vi "lab7.vi"() -> ()   [LabVIEW 2020]
uses:
  <vilib>/measure/NI_MABase.lvlib
  <vilib>/measure/NI_MAPro.lvlib
  <vilib>/gmath/NI_Gmath.lvlib
  <vilib>/Analysis/NI_AALPro.lvlib
  <vilib>/Analysis/2dsp.llb/Power Spectrum (DBL).vi
  <vilib>/Analysis/4window.llb/Blackman Window (DBL).vi
  <vilib>/measure/macond.llb/IIR Filter for 1 Chan.vi
  <vilib>/Analysis/4window.llb/Cosine Tapered Window (DBL).vi
  <vilib>/Analysis/4window.llb/Hamming Window (DBL).vi
  <vilib>/Analysis/4window.llb/Blackman-Harris Window (DBL).vi
  <vilib>/Analysis/3filter.llb/Filter Structure Type.ctl
  <vilib>/Analysis/NI_AALBase.lvlib
panel:
  in  "OK Button":bool
  in  "signal type 2":T1(ring)
  out "Intensity Chart":sgl[][](graph)
  out "Waveform Chart 2":dbl[](graph)
  out "Waveform Chart":dbl[](graph)
  in  "?":bool
  in  "Amplitude 4":dbl=1.0 format="%.2p"
  in  "Window type 2":T2(ring)
  in  "filter structure option 2":T3=10 items=["IIR 2nd Order"=0, "IIR 4th Order"=1, "Auto Select"=10]
  in  "Filter specifications 2":T4={"Topology"=enum."Butterworth", "Type"=enum."Lowpass", "Order"=1, "Lower Fc"=100.0, "Upper Fc"=200.0, "PB Ripple"=1.0, "SB Attenuation"=60.0} {"PB Ripple" format="%0.2f"; "SB Attenuation" format="%0.2f"; "Lower Fc" format="%0.2p"; "Upper Fc" format="%0.2p"}
  out "Filtered 2":waveform(dbl)(graph)
  out "Sig + noise 2":waveform(dbl)(graph)
  in  "Reset Noise 2":bool
  out "Noise 2":waveform(dbl)(graph)
  in  "noise type 2":T5(ring)
  in  "Mean 2":dbl
  in  "Order 2":dbl
  in  "Start freq 2":dbl
  in  "Delta freq 2":dbl
  in  "Amplitude 2":dbl
  out "Signal 2":waveform(dbl)(graph)
  in  "Reset 2":bool
  in  "Offset 2":dbl
  in  "Square duty cycle, %  2":dbl
  in  "Amplitude 3":dbl
  in  "Phase 2":dbl
  in  "Frequncy 2":dbl
  in  "?":T6(tab)
  # "Sine Wave parameters"
  # "Gamma noise parameters"
  # "Poisson noise parameters"
  # "Other Wave-types parameters"
  # "Multitone noise parameters"
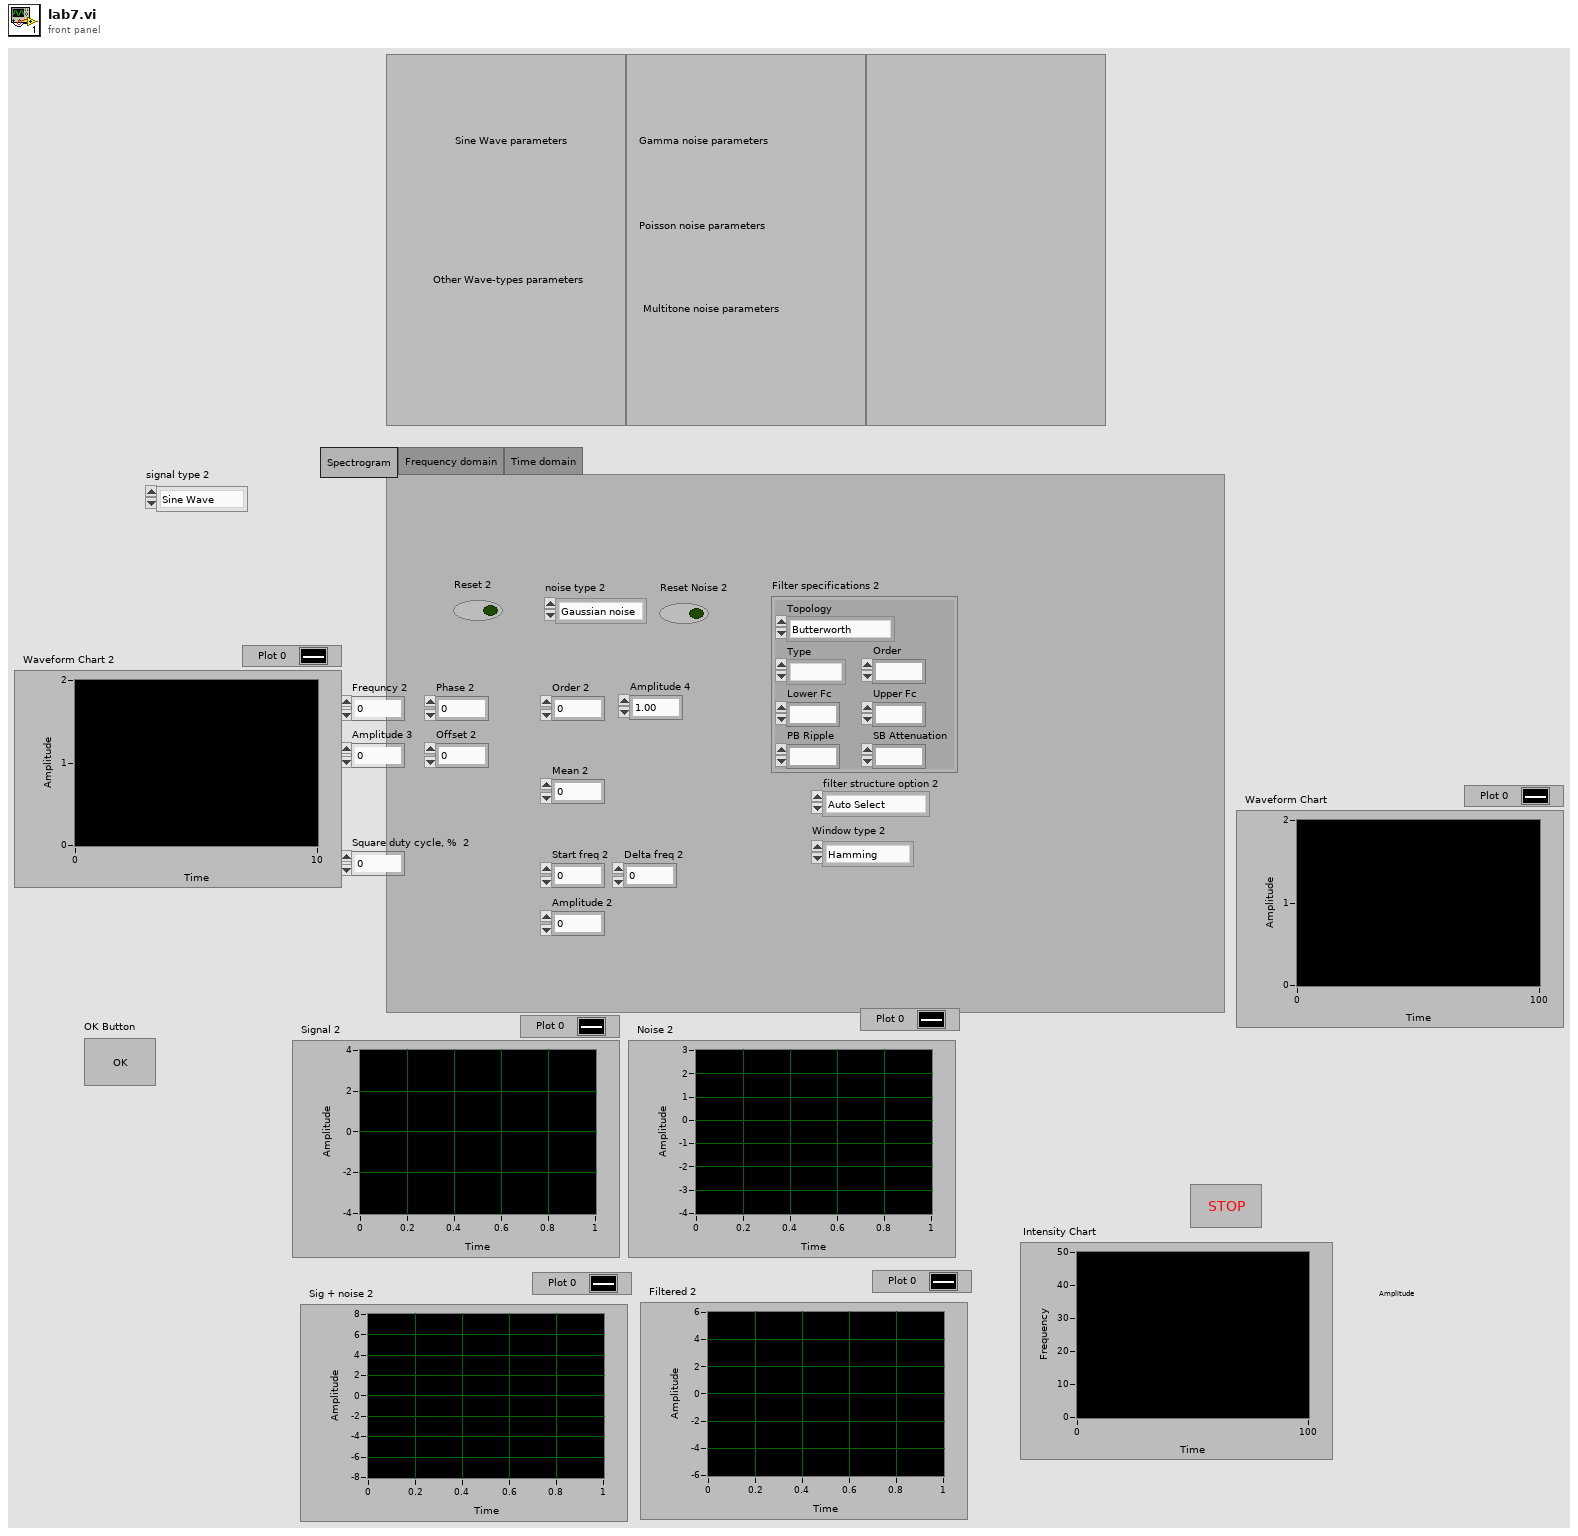
[diagram p1: front panel]
types:
  T1 = enum16{"Sine Wave", "Triangle Wave", "Square Wave", "Sawtooth Wave"}
  T2 = enum16{"Hamming", "Blackman", "Blackman-Harris", "Tapered cos"}
  T3 = typedef "NI_AALBase.lvlib/Filter Structure Type.ctl" = u16
  T4 = cluster{"Topology":enum16{"Off", "Butterworth", "Chebyshev", "Inverse Chebyshev", "Elliptic", "Bessel"}, "Type":enum16{"Lowpass", "Highpass", "Bandpass", "Bandstop"}, "Order":i32, "Lower Fc":dbl, "Upper Fc":dbl, "PB Ripple":dbl, "SB Attenuation":dbl}
  T5 = enum16{"Gaussian noise", "Multitone Noise", "Gamma Noise", "Poisson Noise"}
  T6 = enum32{"Spectrogram", "Frequency domain", "Time domain"}
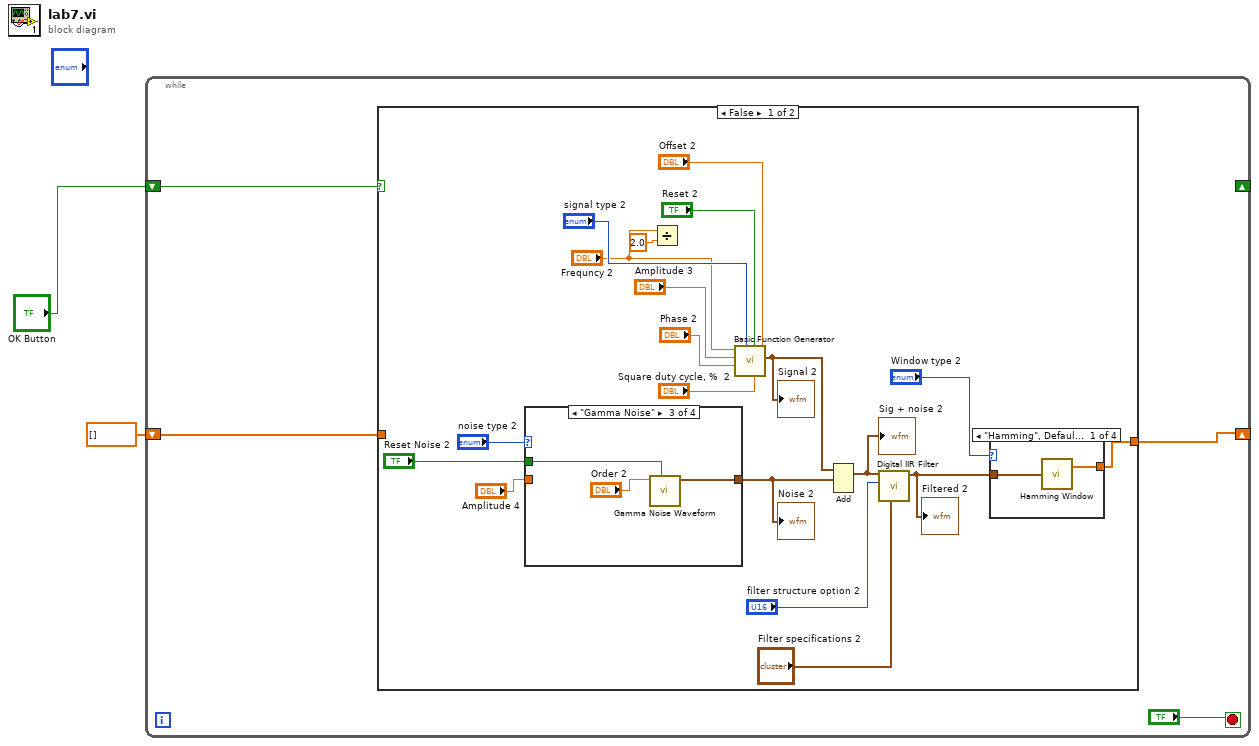
[diagram p0: block diagram]
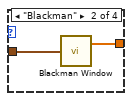
[diagram p2: hidden frame]
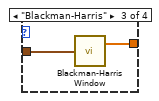
[diagram p3: hidden frame]
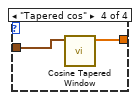
[diagram p4: hidden frame]
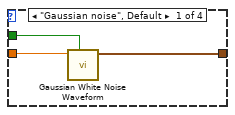
[diagram p5: hidden frame]
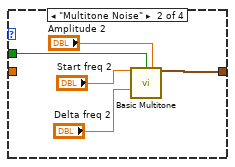
[diagram p6: hidden frame]
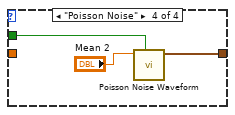
[diagram p7: hidden frame]
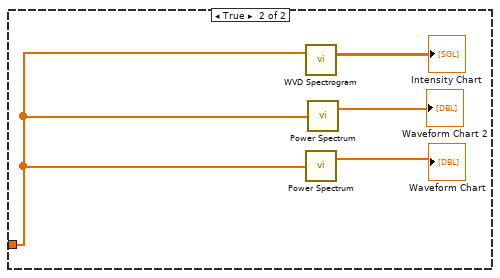
[diagram p8: hidden frame]
diagram:
  n1 = while {
    shift-right: [w4] -> _
    shift-left: dbl[] [] ("Windowed X") -> [w5]
    shift-right: _ -> [_]
    shift-left: "OK Button" -> [w3]
    stop <- "?" stop-if-true
    n2 = case shown="False" w3 {
      tunnel: [w7 _] -> w4
      tunnel: w5 -> [_ w49]
      frame False {
        n3 = case shown="\"Gamma Noise\"" "noise type 2" {
          tunnel: [w36 w40 w43 w45] -> w15
          tunnel: "Reset Noise 2" -> [w35 w41 w42 w47]
          tunnel: "Amplitude 4" -> [w34 _ _ _]
          frame "Gaussian noise", Default {
            n4 = call <vilib>:"Gaussian White Noise Waveform.vi"("reset signal"=w35, "standard deviation"=w34) -> ("signal out"=w36:waveform(dbl))  [unwired: 8 in, 1 out]
          }
          frame "Multitone Noise" {
            n5 = call <vilib>:"Basic Multitone.vi"("start frequency"="Start freq 2", "reset signal"=w41, "amplitude"="Amplitude 2", "delta frequency"="Delta freq 2") -> ("signal out"=w40:waveform(dbl))  [unwired: 8 in, 3 out]
          }
          frame "Gamma Noise" {
            n6 = call <vilib>:"Gamma Noise Waveform.vi"("reset signal"=w42, "order"="Order 2") -> ("signal out"=w43:waveform(dbl))  [unwired: 8 in, 1 out]
          }
          frame "Poisson Noise" {
            n7 = call <vilib>:"Poisson Noise Waveform.vi"("reset signal"=w47, "mean"="Mean 2") -> ("signal out"=w45:waveform(dbl))  [unwired: 8 in, 1 out]
          }
        }
        "Noise 2" <- w15
        n8 = Divide(x="Frequncy 2", y=2.0) -> ()  [unwired: 1 out]
        n9 = call <vilib>:"Basic Function Generator.vi"("offset"="Offset 2", "square wave duty cycle (%)"="Square duty cycle, %  2", "reset signal"="Reset 2", "signal type"="signal type 2", "phase"="Phase 2", "amplitude"="Amplitude 3", "frequency"="Frequncy 2") -> ("signal out"=w12:waveform(dbl))  [unwired: 2 in, 2 out]
        "Signal 2" <- w12
        n10 = Add(1:w15, 2:w12) -> (0:w11:waveform(dbl))  [unwired: 1 in, 1 out]
        "Sig + noise 2" <- w11
        n11 = call-poly <vilib>:"Digital IIR Filter.vi"("IIR filter specifications"="Filter specifications 2", "filter structure option"="filter structure option 2", "signal in"=w11) -> ("signal out"=w9:waveform(dbl))  [unwired: 6 in, 2 out]
        "Filtered 2" <- w9
        n12 = case shown="\"Hamming\", Default" "Window type 2" {
          tunnel: w9 -> [w27 w29 w31 w33]
          tunnel: [w26 w28 w30 w32] -> w7
          frame "Hamming", Default {
            n13 = call-poly <vilib>:"Hamming Window.vi"("X"=w27) -> ("Windowed X"=w26:dbl[])  [unwired: 1 out]
          }
          frame "Blackman" {
            n14 = call-poly <vilib>:"Blackman Window.vi"("X"=w29) -> ("Windowed X"=w28:dbl[])  [unwired: 1 out]
          }
          frame "Blackman-Harris" {
            n15 = call-poly <vilib>:"Blackman-Harris Window.vi"("X"=w31) -> ("Windowed X"=w30:dbl[])  [unwired: 1 out]
          }
          frame "Tapered cos" {
            n16 = call-poly <vilib>:"Cosine Tapered Window.vi"("X"=w33) -> ("Windowed X"=w32:dbl[])  [unwired: 9 in, 1 out]
          }
        }
      }
      frame True {
        n17 = call <vilib>:"WVD Spectrogram.vi"("X"=w49) -> ("WVD Spectrogram {X}"=→"Intensity Chart":sgl[][])  [unwired: 1 in, 1 out]
        n18 = call-poly <vilib>:"Power Spectrum.vi"("X"=w49) -> ("Power Spectrum"=→"Waveform Chart":dbl[])  [unwired: 1 out]
        n19 = call-poly <vilib>:"Power Spectrum.vi"("X"=w49) -> ("Power Spectrum"=→"Waveform Chart 2":dbl[])  [unwired: 1 out]
      }
    }
  }
